vi "Load Script.vi"(7 "Script Name":string="TSB_Script", 8 "error in (no error)":errorcluster caption="错误输入（无错误）", 10 "Script":string, 11 "2601B 输入":refnum<class "2601B.lvclass">) -> (0 "error out":errorcluster caption="错误输出", 3 "2601B 输出":refnum<class "2601B.lvclass">)   [LabVIEW 2020, in "2601B.lvclass"]
uses:
  2601B.lvclass
  2601B.lvclass/2601B.ctl
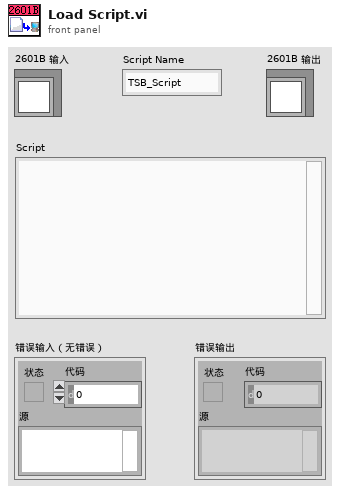
[diagram p1: front panel]
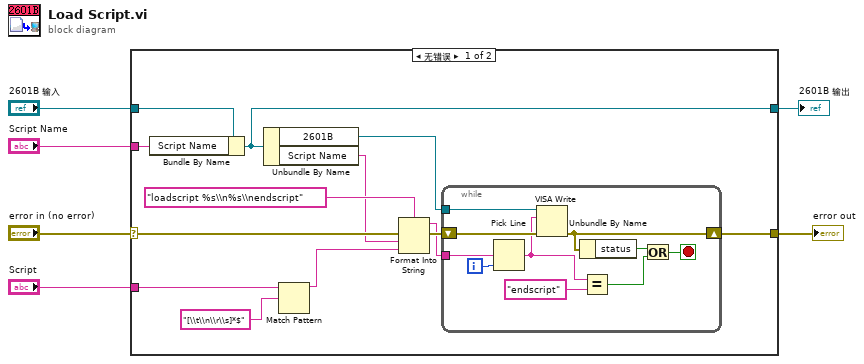
[diagram p0: block diagram]
diagram:
  n1 = case shown="无错误" "error in (no error)" {
    selector: "error in (no error)" -> [w14 w31]
    tunnel: [w13 w31] -> w5
    tunnel: [w12 w30] -> w3
    tunnel: "2601B 输入" -> [w16 w30]
    tunnel: "Script" -> [w8 _]
    tunnel: "Script Name" -> [w11 _]
    frame No Error {
      n2 = Bundle By Name(cluster=w16, "Script Name"=w11) -> (w12:refnum<class "2601B.lvclass">)
      n3 = Unbundle By Name(w12) -> ("2601B"=w15:refnum<visa-resource-name>, "Script Name"=w10:string)
      n4 = Match Pattern(string=w8, regular expression="[\\t\\n\\r\\s]*$") -> (before substring=w7:string)  [unwired: 1 in, 3 out]
      n5 = Format Into String(format string="loadscript %s\\n%s\\nendscript", error in=w14, w10, w7) -> (resulting string=w17:string, error out=w18:errorcluster)  [unwired: 1 in]
      n6 = while {
        tunnel: w15 -> [w28]
        shift-right: [w22] -> w13
        shift-left: w18 -> [w29]
        tunnel: w17 -> [w26]
        i -> [w25]
        stop <- w20 stop-if-true
        n7 = Pick Line(multi-line string=w26, line index=w25) -> (output string=w21:string)  [unwired: 1 out]
        n8 = VISA Write(VISA resource name=w28, write buffer=w21, error in (no error)=w29) -> (error out=w22:errorcluster)  [unwired: 2 out]
        n9 = Unbundle By Name(w22) -> ("status"=w24:bool)
        n10 = Equal?(x=w21, y="endscript") -> (x = y?=w23:bool)
        n11 = Or(x=w24, y=w23) -> (x .or. y?=w20:bool)
      }
    }
    frame Error {
    }
  }
  "error out" <- w5
  "2601B 输出" <- w3
